vi "DrawHints.vi"(9 "Hints":bool[](array[boolean]), 10 "rect":T1, 11 "picture in":picture) -> (3 "picture out":picture)   [LabVIEW 2021, in "Cell.lvclass"]
uses:
  Cell.lvclass
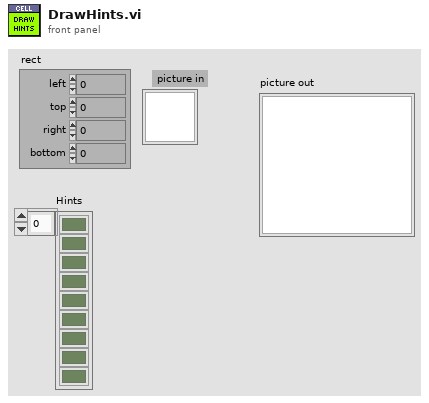
[diagram p1: front panel]
types:
  T1 = cluster{"left":i16, "top":i16, "right":i16, "bottom":i16}
  T2 = cluster{"Width":i16, "Style":enum32{"Solid", "Dash", "Dot", "DashDot", "DashDotDot"}}
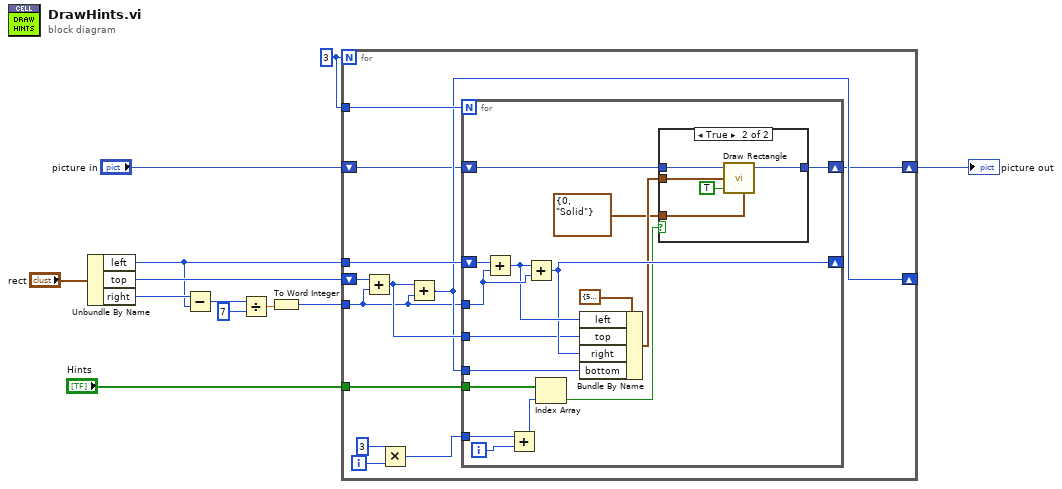
[diagram p0: block diagram]
diagram:
  w7 = 3
  n1 = Unbundle By Name("rect") -> ("left"=w4:i16, "top"=w5:i16, "right"=w11:i16)
  n2 = Subtract(x=w11, y=w4) -> (x-y=w10:i16)
  n3 = Divide(x=w10, y=i16 7) -> (x/y=w8:dbl)
  n4 = To Word Integer(number=w8) -> (16bit integer=w3:i16)
  n5 = for {
    N: w7 -> [_]
    tunnel: w7 -> [w24]
    tunnel: "Hints" -> [w23]
    shift-right: [w16] -> _
    shift-left: w5 -> [w19]
    tunnel: w4 -> [w18]
    tunnel: w3 -> [w13]
    shift-right: [w14] -> w2
    shift-left: "picture in" -> [w15]
    i -> [w22]
    n6 = Add(x=w19, y=w13) -> (x+y=w17:i16)
    n7 = Multiply(x=3, y=w22) -> (x*y=w20:i32)
    n8 = Add(x=w17, y=w13) -> (x+y=w16:i16)
    n9 = for {
      N: w24 -> [_]
      tunnel: w23 -> [w38]
      tunnel: w20 -> [w39]
      shift-right: [w32] -> _
      shift-left: w18 -> [w36]
      tunnel: w13 -> [w35]
      tunnel: w17 -> [w31]
      tunnel: w16 -> [w30]
      shift-right: [w27] -> w14
      shift-left: w15 -> [w28]
      i -> [w40]
      n10 = Add(x=w36, y=w35) -> (x+y=w33:i16)
      n11 = Add(x=w39, y=w40) -> (x+y=w37:i32)
      n12 = Add(x=w33, y=w35) -> (x+y=w32:i16)
      n13 = Index Array(array=w38, index=w37) -> (element=w29:bool)
      n14 = Bundle By Name(cluster=T1 {"left"=5, "top"=5, "right"=100, "bottom"=100} ("rect"), "left"=w33, "top"=w31, "right"=w32, "bottom"=w30) -> (w26:T1)
      n15 = case shown="True" w29 {
        tunnel: w28 -> [w41 w46]
        tunnel: [w41 w45] -> w27
        tunnel: w26 -> [_ w44]
        tunnel: T2 {"Width"=0, "Style"=enum."Solid"} ("pen") -> [_ w42]
        frame False {
        }
        frame True {
          n16 = call <vilib>:"Draw Rectangle.vi"("picture"=w46, "rect"=w44, "fill?(F)"=TRUE, "pen"=w42) -> ("new picture"=w45:picture)  [unwired: 5 in]
        }
      }
    }
  }
  "picture out" <- w2
